vi "Auto Drive.vi"(0 "Distance Target":dbl, 2 "Strafe Target":dbl, 3 "Y Speed":dbl, 5 "Z Speed":dbl, 7 "Async?":dbl) -> (19 "Finished?":bool)   [LabVIEW 2016]
uses:
  Common Code/Drivetrain Mode.ctl
  Robot Global Data.vi
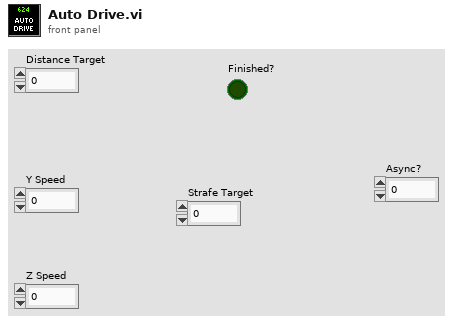
[diagram p1: front panel]
types:
  T1 = typedef "Drivetrain Mode.ctl" = enum16{"Manual", "Gyro Steer", "Distance Drive", "Translate Drive", "Goal Vision Align", "PID Drive"}
  T2 = typedef "Drivetrain Status Cluster.ctl" = cluster{"Drivetrain Mode":enum16{"Manual", "Gyro Steer"}, "Y (Throttle)":dbl, "X (Steer)":dbl, "Z (Strafe)":dbl, "Heading Target":dbl, "Center Piston Down?":bool, "Traction?":bool, "Gyro Steer Finished?":bool, "Distance Drive Finished?":bool, "Gyro":dbl, "Distance Target":dbl, "Y Max Output":dbl, "Y Min Output":dbl, "X Max Output":dbl, "X Min Output":dbl, "Z Max Output":dbl, "Z Min Output":dbl, "Translation Target":dbl, "Translation Drive Finished?":bool, "PID Auto Drive Finished?":bool, "Brake?":bool, "Vision Aligned?":bool}
  T3 = typedef "Drivetrain Command Cluster.ctl" = cluster{"Drivetrain Mode":T1, "Heading Target":dbl, "Turn Power":dbl, "Y Power":dbl, "Center Piston Down?":bool, "Traction?":bool, "Strafe Power":dbl, "Zero Gyro":bool, "Distance Target":dbl, "Strafe Correct":bool, "Y Max Output":dbl, "Y Min Output":dbl, "X Max Output":dbl, "X Min Output":dbl, "Z Max Output":dbl, "Z Min Output":dbl, "Z Target":dbl, "Brake?":bool}
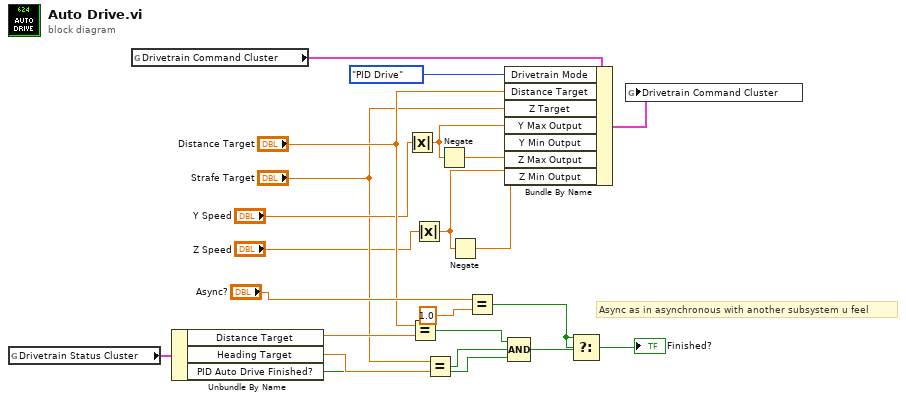
[diagram p0: block diagram]
diagram:
  # "Async as in asynchronous with another subsystem u feel"
  n1 = global read "Robot Global Data.vi" "Drivetrain Status Cluster"() -> (w18:T2)
  n2 = global read "Robot Global Data.vi" "Drivetrain Command Cluster"() -> (w14:T3)
  n3 = Unbundle By Name(w18) -> ("Distance Target"=w17:dbl, "Heading Target"=w8:dbl, "PID Auto Drive Finished?"=w7:bool)
  n4 = Absolute Value(x="Y Speed") -> (abs(x)=w4:dbl)
  n5 = Equal?(x="Distance Target", y=w17) -> (x = y?=w16:bool)
  n6 = Absolute Value(x="Z Speed") -> (abs(x)=w2:dbl)
  n7 = Equal?(x="Strafe Target", y=w8) -> (x = y?=w6:bool)
  n8 = Negate(x=w4) -> (-x=w5:dbl)
  n9 = Negate(x=w2) -> (-x=w1:dbl)
  n10 = Equal?(x="Async?", y=1.0) -> (x = y?=w20:bool)
  n11 = Bundle By Name(cluster=w14, "Drivetrain Mode"=Drivetrain_Mode."PID Drive", "Distance Target"="Distance Target", "Z Target"="Strafe Target", "Y Max Output"=w4, "Y Min Output"=w5, "Z Max Output"=w2, "Z Min Output"=w1) -> (w13:T3)
  n12 = Compound Arithmetic op=AND(w16, w6, w7) -> (w15:bool)
  n13 = Select(t=w20, s=w20, f=w15) -> (s? t:f=→"Finished?":bool)
  n14 = global write "Robot Global Data.vi" "Drivetrain Command Cluster"(w13) -> ()
